vi "Strat-parse-load.vi"(8 "error in":errorcluster, 10 "Info JSON - rel path":path=path "../strat_cl1_info_dict.json", 11 "Strategy JSON - rel path":path=path "../strat_cl1_dict.json") -> (0 "error out":errorcluster, 2 "Regional clusters":T1[](array[typedef]), 3 "Index array":i32[](array[numeric]))   [LabVIEW 2016]
uses:
  Strategy_regional_cluster.ctl
  Strategy_regional_set.ctl
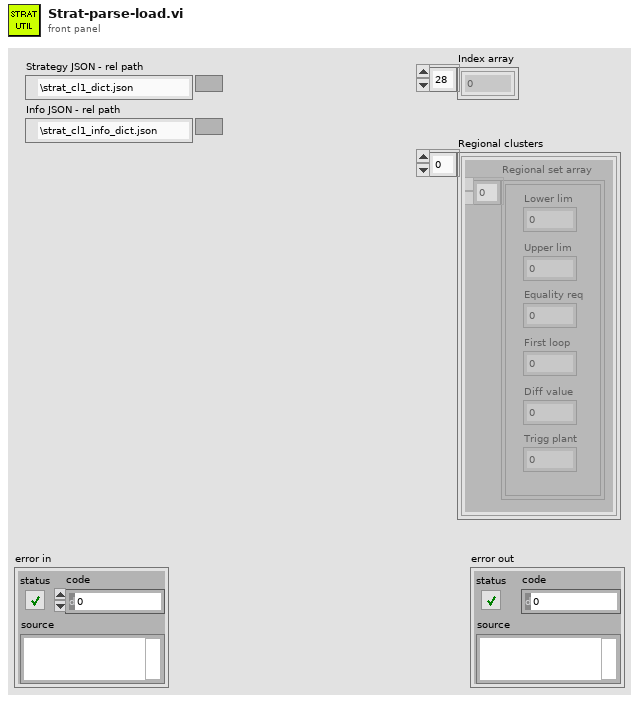
[diagram p1: front panel]
types:
  T1 = typedef "Strategy_regional_cluster.ctl" = cluster{"Regional set array":T2[]}
  T2 = typedef "Strategy_regional_set.ctl" = cluster{"Lower lim":i32, "Upper lim":i32, "Equality req":i32, "First loop":i32, "Diff value":i32, "Trigg plant":i32}
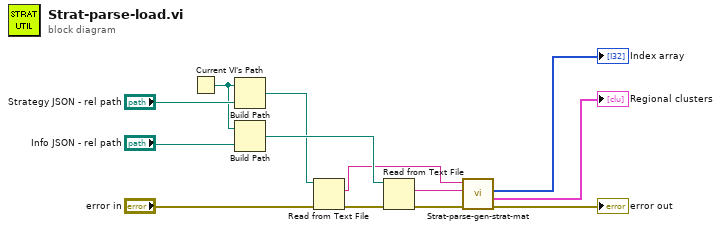
[diagram p0: block diagram]
diagram:
  n1 = Current VI's Path() -> (path=w12:path)
  n2 = Build Path(base path=w12, name or relative path="Strategy JSON - rel path") -> (appended path=w9:path)
  n3 = Build Path(base path=w12, name or relative path="Info JSON - rel path") -> (appended path=w10:path)
  n4 = Read from Text File(file (use dialog)=w9, error in="error in") -> (text=w5:string, error out=w6:errorcluster)  [unwired: 2 in, 2 out]
  n5 = Read from Text File(file (use dialog)=w10, error in=w6) -> (text=w8:string, error out=w4:errorcluster)  [unwired: 2 in, 2 out]
  n6 = call "Strat-parse-gen-strat-mat.vi"("error in (no error)"=w4, "Info JSON"=w8, "Strategy JSON"=w5) -> ("error out"=→"error out":errorcluster, "Regional clusters"=→"Regional clusters":T1[], "Index array"=→"Index array":i32[])  [unwired: 5 in, 1 out]
